vi "Joystick_control.vi"() -> ()   [LabVIEW 2019]
uses:
  <vilib>/MakerHub/LINX/Public/Peripherals/Analog/Analog Read 1 Chan.vi
  <vilib>/MakerHub/LINX/Public/Peripherals/Digital/Digital Write 1 Chan.vi
  <vilib>/MakerHub/LINX/Public/Peripherals/Analog/Analog Read N Chans.vi
  <vilib>/MakerHub/LINX/Public/Peripherals/Digital/Digital Write N Chans.vi
  <vilib>/MakerHub/LINX/Private/Local IO/LinxAnalogRead.vi
  <vilib>/MakerHub/LINX/Public/Utilities/Check Channel.vi
  <vilib>/MakerHub/LINX/Private/Local IO/LinxDigitalWrite.vi
  <vilib>/MakerHub/LINX/Public/Utilities/Open Serial.vi
  <vilib>/MakerHub/LINX/Private/Utilties/Generate Error.vi
  <vilib>/MakerHub/LINX/LMH-LINX.lvlib
panel:
  in  "Serial Port":refnum<visa-resource-name>="N/A"
  in  "stop":bool
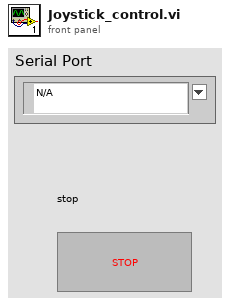
[diagram p1: front panel]
types:
  T1 = typedef "LMH-LINX.lvlib/LINX Ref.ctl" = cluster{"IO":T2, "Interface":T3, "LINX Device Config":T4}
  T2 = typedef "LMH-LINX.lvlib/Platform.ctl" = enum16{"Remote", "Local"}
  T3 = typedef "LMH-LINX.lvlib/Interface.ctl" = enum16{"Serial", "TCP"}
  T4 = typedef "LMH-LINX.lvlib/Device.lvlib/LINX Device Config.ctl" = cluster{"Interface":T3, "COM Port":refnum<visa-resource-name>, "TCP Configuration":T5, "Device Family":u8, "Device ID":u8, "Device Name":string, "TCP Ref":refnum<k5>, "Channels":T6}
  T5 = typedef "LMH-LINX.lvlib/Device.lvlib/TCP Config.ctl" = cluster{"IP Address":string, "Port":u16}
  T6 = typedef "LMH-LINX.lvlib/Channels.ctl" = cluster{"DI":u8[], "DO":u8[], "AI":u8[], "AO":u8[], "PWM":u8[], "QE":u8[], "UART":u8[], "I2C 2":u8[], "SPI":u8[], "CAN":u8[], "Servo":u8[], "AI Ref (V)":dbl, "AI Resolution (Bits)":u8, "AO Ref (V)":dbl, "AO Resolution (Bits)":u8}
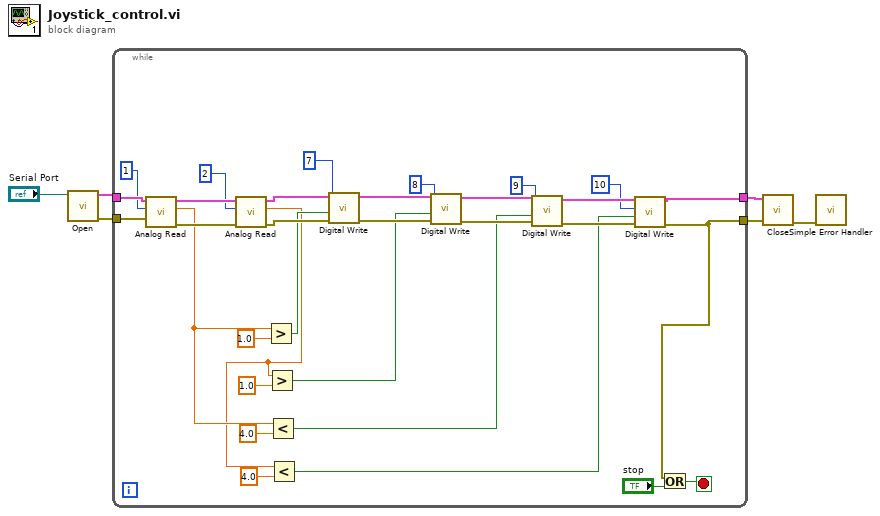
[diagram p0: block diagram]
diagram:
  n1 = call-poly <vilib>:"Open.vi"("Serial Port"="Serial Port") -> ("Error Out"=w3:errorcluster, "LINX Resource"=w6:T1)  [unwired: 8 in, 1 out]
  n2 = while {
    tunnel: w6 -> [w36]
    tunnel: [w8] -> w5
    tunnel: w3 -> [w35]
    tunnel: [w7] -> w2
    stop <- w37 stop-if-true
    n3 = call-poly <vilib>:"Analog Read.vi"("Error In"=w35, "Analog Channel"=u8 1, "LINX Resource"=w36) -> ("Error Out"=w22:errorcluster, "Voltage"=w14:dbl, "LINX Resource"=w24:T1)  [unwired: 5 in, 1 out]
    n4 = call-poly <vilib>:"Analog Read.vi"("Error In"=w22, "Analog Channel"=u8 2, "LINX Resource"=w24) -> ("Error Out"=w21:errorcluster, "Voltage"=w13:dbl, "LINX Resource"=w23:T1)  [unwired: 5 in, 1 out]
    n5 = Greater?(x=w14, y=1.0) -> (0:w18:bool)
    n6 = Greater?(x=w13, y=1.0) -> (0:w17:bool)
    n7 = Less?(x=w14, y=4.0) -> (x < y?=w16:bool)
    n8 = Less?(x=w13, y=4.0) -> (x < y?=w15:bool)
    n9 = call-poly <vilib>:"Digital Write.vi"("Error In"=w21, "Output Value"=w18, "DO Channel"=u8 7, "LINX Resource"=w23) -> ("Error Out"=w31:errorcluster, "LINX Resource"=w34:T1)  [unwired: 6 in]
    n10 = call-poly <vilib>:"Digital Write.vi"("Error In"=w31, "Output Value"=w17, "DO Channel"=u8 8, "LINX Resource"=w34) -> ("Error Out"=w30:errorcluster, "LINX Resource"=w33:T1)  [unwired: 6 in]
    n11 = call-poly <vilib>:"Digital Write.vi"("Error In"=w30, "Output Value"=w16, "DO Channel"=u8 9, "LINX Resource"=w33) -> ("Error Out"=w29:errorcluster, "LINX Resource"=w32:T1)  [unwired: 6 in]
    n12 = call-poly <vilib>:"Digital Write.vi"("Error In"=w29, "Output Value"=w15, "DO Channel"=u8 10, "LINX Resource"=w32) -> ("Error Out"=w7:errorcluster, "LINX Resource"=w8:T1)  [unwired: 6 in]
    n13 = Or(x=w7, y="stop") -> (x .or. y?=w37:bool)
  }
  n14 = call <vilib>:"Close.vi"("Error In"=w2, "LINX Resource"=w5) -> ("Error Out"=w1:errorcluster)  [unwired: 9 in]
  n15 = call <vilib>:"Simple Error Handler.vi"("error in (no error)"=w1) -> ()  [unwired: 4 in, 5 out]
